vi "Teleop-System-Dash-Write.vi"   [LabVIEW 2019]
uses:
  Teleop-System-Globals.vi
  <vilib>/Rock Robotics/Network Tables/NT Write Numeric Array.vi
  <vilib>/Rock Robotics/Network Tables/NT Write Boolean Array.vi
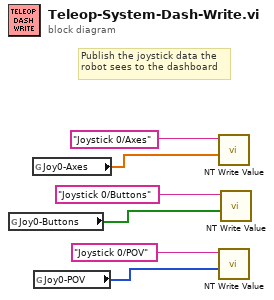
[diagram p0: block diagram]
diagram:
  # "Publish the joystick data the\nrobot sees to the dashboard"
  n1 = global read "Teleop-System-Globals.vi" "Joy0-Buttons"() -> (w3:bool[])
  n2 = global read "Teleop-System-Globals.vi" "Joy0-Axes"() -> (w4:dbl[])
  n3 = global read "Teleop-System-Globals.vi" "Joy0-POV"() -> (w1:i32[])
  n4 = call-poly <vilib>:"NT Write Value.vi"("Numeric Array"=w4, "Name"="Joystick 0/Axes") -> ()  [unwired: 9 in, 1 out]
  n5 = call-poly <vilib>:"NT Write Value.vi"("Numeric Array"=w1, "Name"="Joystick 0/POV") -> ()  [unwired: 9 in, 1 out]
  n6 = call-poly <vilib>:"NT Write Value.vi"("Boolean Array"=w3, "Name"="Joystick 0/Buttons") -> ()  [unwired: 9 in, 1 out]
